vi "Launch VF Device Selection Dialog.vi"(8 "error in":errorcluster, 11 "Master Controller in":refnum<class "EMS User Interface.lvclass">) -> (0 "error out":errorcluster, 3 "Master Controller out":refnum<class "EMS User Interface.lvclass">)   [LabVIEW 2018, in "EMS User Interface Actor.lvlib" / "EMS User Interface.lvclass"]
uses:
  EMS User Interface.lvclass
  C:/Users/Administrator/Desktop/LabVIEW EMS/EMS Generic Actor/EMS Generic/EMS Generic.lvclass
  C:/Program Files (x86)/National Instruments/LabVIEW 2018/vi.lib/ActorFramework/Actor/Actor.lvclass
  Dialog Actors/VF Device Selection Actor/VF Device Selection/VF Device Selection.lvclass
  EMS Generic Actor/EMS Generic/EMS Generic.lvclass/EMS Generic.ctl
  EMS User Interface.lvclass/EMS User Interface.ctl
  Dialog Actors/VF Device Selection Actor/VF Device Selection Messages/Update Device List Msg/Update Device List Msg.lvclass/Update Device List Msg.ctl
  <vilib>/ActorFramework/Message Enqueuer/Message Enqueuer.lvclass/Message Enqueuer.ctl
  <vilib>/ActorFramework/Message Enqueuer/Enqueue.vi
  Dialog Actors/VF Device Selection Actor/VF Device Selection Messages/Update Device List Msg/Update Device List Msg.lvclass
  C:/Program Files (x86)/National Instruments/LabVIEW 2018/vi.lib/ActorFramework/Message/Message.lvclass
  Global Variables/Global Variables.vi
  <vilib>/ActorFramework/Message Priority Queue/Priority Enqueue.vi
  <vilib>/ActorFramework/Actor/Actor.lvclass
  EMS Generic Actor/EMS Generic/EMS Generic.lvclass
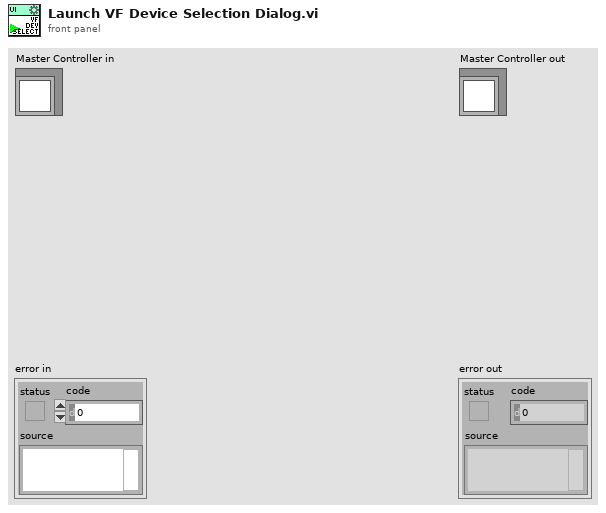
[diagram p1: front panel]
types:
  T1 = typedef "CSEISMIC DDS.lvlib/CSEISMIC DDS.lvclass/DeviceID.ctl" = string
  T2 = typedef "EMS Generic Actor.lvlib/EMS Generic.lvclass/Data Type DVRs.ctl" = cluster{"IED_Status":refnum<data-value>, "IED_Status_0":refnum<data-value>, "DER_Measurement":refnum<data-value>, "DER_Info":refnum<data-value>, "DER_Status":refnum<data-value>, "ES_Measurement":refnum<data-value>, "ES_Info":refnum<data-value>, "PV_Info":refnum<data-value>, "SmartRelay_Info":refnum<data-value>, "SmartRelay_Measurement":refnum<data-value>, "Meter_Info":refnum<data-value>, "Meter_Measurement":refnum<data-value>, "HVAC_Status":refnum<data-value>, "HVAC_Measurement":refnum<data-value>, "PriceData_RealTime":refnum<data-value>, "PriceData_Demand":refnum<data-value>, "PriceData_Energy":refnum<data-value>, "ForecastData_Long":refnum<data-value>, "ForecastData_Short":refnum<data-value>, "DER_Control":refnum<data-value>, "DER_SetPointF":refnum<data-value>, "DER_SetPointP":refnum<data-value>, "DER_SetPointQ":refnum<data-value>, "DER_SetPointPF":refnum<data-value>, "DER_SetPointV":refnum<data-value>, "PV_setCurtailment":refnum<data-value>, "PV_setRampRate":refnum<data-value>, "Relay_Control":refnum<data-value>, "Load_Control":refnum<data-value>, "HVAC_Control":refnum<data-value>, "Generator_Info":refnum<data-value>, "ForecastData_Long_Backup":refnum<data-value>, "PriceData_RealTime_Backup":refnum<data-value>}
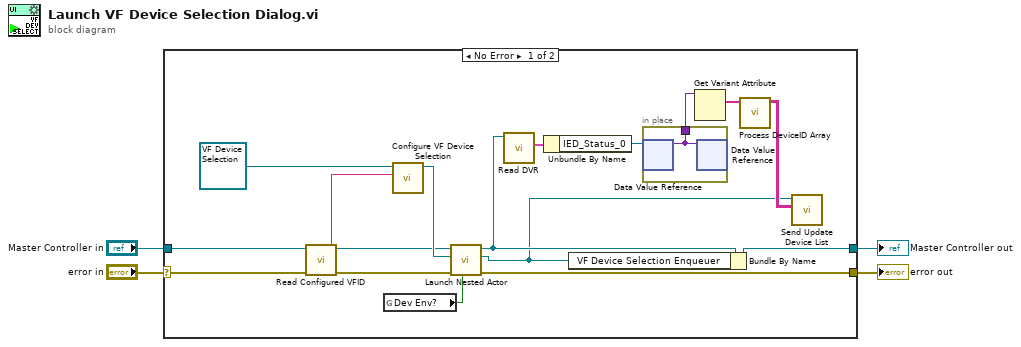
[diagram p0: block diagram]
diagram:
  n1 = case shown="No Error" "error in" {
    selector: "error in" -> [w14 w24]
    tunnel: [w20 w24] -> w3
    tunnel: [w19 w23] -> w1
    tunnel: "Master Controller in" -> [w16 w23]
    frame No Error {
      n2 = call "Read Configured VFID.vi"("error in"=w14, "EMS Generic in"=w16) -> ("error out"=w13:errorcluster, "VFID"=w15:T1, "EMS Generic out"=w12:refnum<class "EMS User Interface.lvclass">)  [unwired: 7 in]
      n3 = global read "Global Variables.vi" "Dev Env?"() -> (w18:bool)
      n4 = call "Configure VF Device Selection.vi"("VF DeviceID"=w15, "VF Device Selection in"=refnum<class "VF Device Selection.lvclass"> refnum ("VF Device Selection Actor.lvlib:VF Device Selection.lvclass")) -> ("VF Device Selection out"=w21:refnum<class "VF Device Selection.lvclass">)  [unwired: 9 in]
      n5 = call <vilib>:"Launch Nested Actor.vi"("Open Actor Core front panel? (F)"=w18, "error in (no error)"=w13, "Nested Actor"=w21, "Caller Actor in"=w12) -> ("error out"=w20:errorcluster, "Nested Actor's Enqueuer"=w5:refnum<class "Message Enqueuer.lvclass">, "Caller Actor out"=w7:refnum<class "EMS User Interface.lvclass">)  [unwired: 5 in]
      n6 = call "Read DVR.vi"("EMS Generic in"=w7) -> ("DVR"=w8:T2)  [unwired: 9 in, 1 out]
      n7 = Unbundle By Name(w8) -> ("IED_Status_0"=w9:refnum<data-value>)
      n8 = Bundle By Name(cluster=w7, "VF Device Selection Enqueuer"=w5) -> (w19:refnum<class "EMS User Interface.lvclass">)
      n9 = in-place {
        in-place-border: [w22] -> w10
        n10 = in-place-dvr #1(w9) -> (w22:variant)  [unwired: 1 out]
        n11 = in-place-dvr #1(w22) -> ()  [unwired: 2 out]
      }
      n12 = Get Variant Attribute(Variant=w10) -> (names=w11:string[])  [unwired: 3 in, 3 out]
      n13 = call "Process DeviceID Array.vi"("DeviceID Array"=w11) -> ("Array"=w6:T1[][])  [unwired: 9 in, 1 out]
      n14 = call "Send Update Device List.vi"("Device Table Strings"=w6, "Message Enqueuer"=w5) -> ()  [unwired: 8 in, 2 out]
    }
    frame Error {
    }
  }
  "error out" <- w3
  "Master Controller out" <- w1
